vi "get_rotation.vi"(8 "error in (no error)":errorcluster, 11 "TrajectoryMH100122AODRAPS in":refnum<class "TrajectoryMH100122AODRAPS.lvclass">) -> (0 "error out":errorcluster, 1 "x angle (tilting angle, phi)":dbl[unit], 2 "z angle (rotation angle, phi)":dbl[unit], 3 "TrajectoryMH100122AODRAPS out":refnum<class "TrajectoryMH100122AODRAPS.lvclass">)   [LabVIEW 2010, in "TrajectoryMH100122AODRAPS.lvclass"]
uses:
  TrajectoryMH100122AODRAPS.lvclass
  TrajectoryMH100122AODRAPS.lvclass/TrajectoryMH100122AODRAPS.ctl
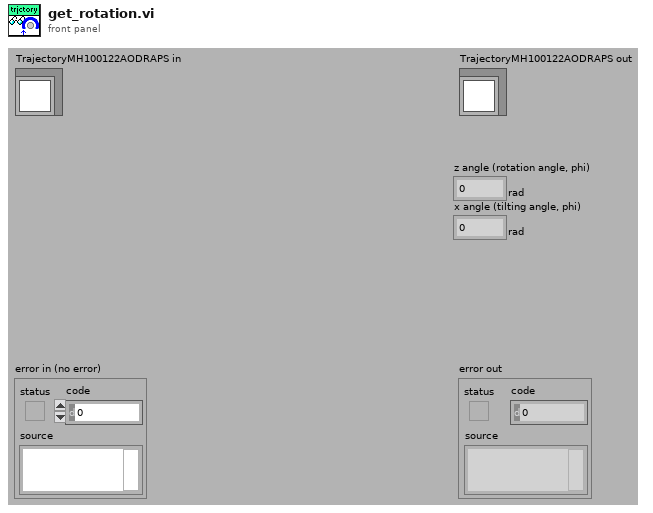
[diagram p1: front panel]
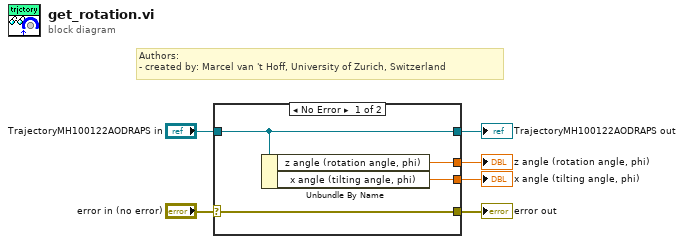
[diagram p0: block diagram]
diagram:
  # "Authors: \n- created by: Marcel van 't Hoff, University of Zurich, Switzerland"
  n1 = case shown="No Error" "error in (no error)" {
    selector: "error in (no error)" -> [w10 w12]
    tunnel: [w10 w12] -> w5
    tunnel: [w9 w11] -> w3
    tunnel: "TrajectoryMH100122AODRAPS in" -> [w9 w11]
    tunnel: [w8 _] -> w2
    tunnel: [w7 _] -> w1
    frame No Error {
      n2 = Unbundle By Name(w9) -> ("z angle (rotation angle, phi)"=w8:dbl[unit], "x angle (tilting angle, phi)"=w7:dbl[unit])
    }
    frame Error {
    }
  }
  "error out" <- w5
  "TrajectoryMH100122AODRAPS out" <- w3
  "z angle (rotation angle, phi)" <- w2
  "x angle (tilting angle, phi)" <- w1
